vi "List property names and values.vi"(2 "Metadata":T1, 4 "Prev eindex":i32, 5 "error in (no error)":errorcluster) -> (16 "List of property names":string, 18 "Last index":i32, 19 "error out":errorcluster)   [LabVIEW 2019, in "metadata.lvclass"]
uses:
  metadata.lvclass
  Metadata output --cluster.ctl
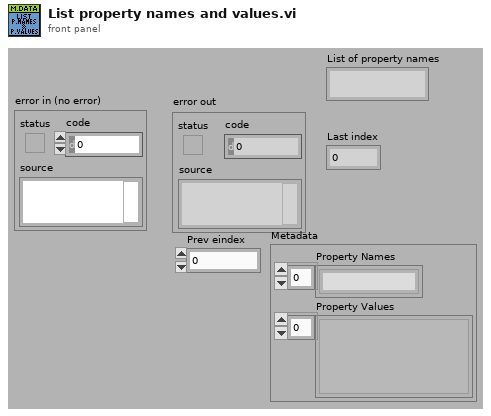
[diagram p1: front panel]
types:
  T1 = typedef "metadata.lvclass/Metadata output --cluster.ctl" = cluster{"Property Names":string[], "Property Values":variant[]}
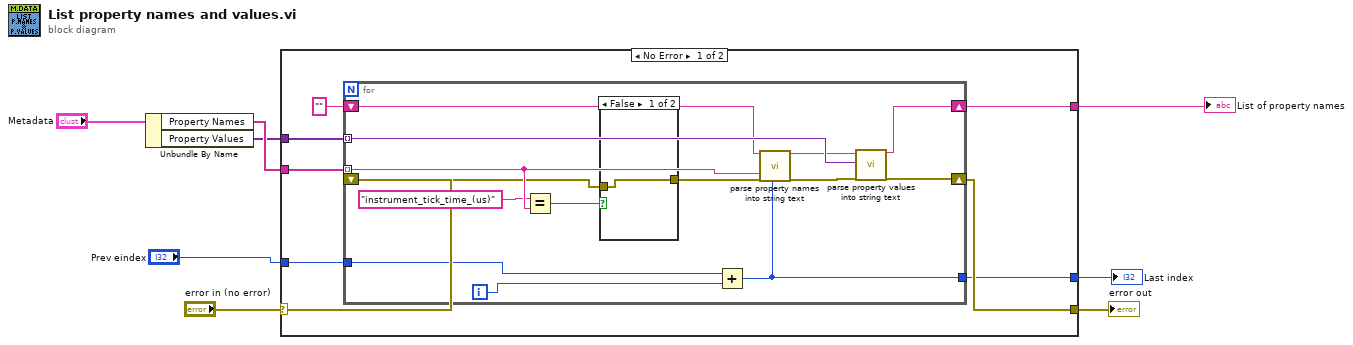
[diagram p0: block diagram]
diagram:
  n1 = Unbundle By Name("Metadata") -> ("Property Names"=w5:string[], "Property Values"=w4:variant[])
  n2 = case shown="No Error" "error in (no error)" {
    selector: "error in (no error)" -> [w14 w34]
    tunnel: [w13 w34] -> w7
    tunnel: w5 -> [w16 _]
    tunnel: [w12 _] -> w2
    tunnel: w4 -> [w11 _]
    tunnel: "Prev eindex" -> [w10 w33]
    tunnel: [w9 w33] -> w1
    frame No Error {
      n3 = for {
        tunnel: w16 -> [w21] mode=indexing
        shift-right: [w28] -> w12
        shift-left: "" ("String in") -> [w24]
        shift-right: [w29] -> w13
        shift-left: w14 -> [w18]
        tunnel: w11 -> [w27] mode=indexing
        tunnel: w10 -> [w26]
        tunnel: [w22] -> w9
        i -> [w25]
        n4 = Equal?(x="instrument_tick_time_(us)", y=w21) -> (x = y?=w19:bool)
        n5 = case shown="False" w19 {
          tunnel: w18 -> [w31 w32]
          tunnel: [w31 w32] -> w17
          frame False {
          }
          frame True {
          }
        }
        n6 = Add(x=w26, y=w25) -> (x+y=w22:i32)
        n7 = call "parse property names into string text.vi"("String in"=w24, "Property names"=w21, "error in (no error)"=w17, "Counter"=w22) -> ("String out"=w23:string, "error out"=w30:errorcluster)  [unwired: 14 in]
        n8 = call "parse property values into string text.vi"("String in"=w23, "Property value"=w27, "error in (no error)"=w30) -> ("String out"=w28:string, "error out"=w29:errorcluster)  [unwired: 15 in]
      }
    }
    frame Error {
    }
  }
  "error out" <- w7
  "List of property names" <- w2
  "Last index" <- w1
